vi "FrameToTag(scalar)__slk_mt.vi"(8 "error in (no error)":errorcluster, 10 "frame":string, 11 "string adapter in":refnum<class "StringAdapter__slk_mt.lvclass">) -> (0 "error out":errorcluster, 2 "tag":string, 3 "string adapter out":refnum<class "StringAdapter__slk_mt.lvclass">)   [LabVIEW 2015, in "StringAdapter__slk_mt.lvclass"]
doc: "Converts case frame name to tree control tag."
uses:
  StringAdapter__slk_mt.lvclass
panel:
  # "FrameToTag(scalar)__slk_mt.vi\nConverts case frame name to tree control tag.\n\nNOTICE -- YOU MUST LEAVE THIS NOTICE IN PLACE.\n\nCopyright (c) 2011, LIANG LIU Shawn.Liu.cn@gmail.com\nAll rights reserved.\n\nRedistribution and use in source and binary forms, with or without modification, are permitted provided that the following conditions are met:\n-Redistributions of source code must retain the above copyright notice, this list of conditions and the following disclaimer.\n-Redistributions in binary form must reproduce the above copyright notice, this list of conditions and the following disclaimer in the documentation and/or other materials provided with the distribution.\n-Neither the name of the eLp nor the names of its contributors may be used to endorse or promote products derived from this software without specific prior written permission.\n\nTHIS SOFTWARE IS PROVIDED BY THE COPYRIGHT HOLDERS AND CONTRIBUTORS \"AS IS\" AND ANY EXPRESS OR IMPLIED WARRANTIES, INCLUDING, BUT NOT LIMITED TO, THE IMPLIED WARRANTIES OF MERCHANTABILITY AND FITNESS FOR A PARTICULAR PURPOSE ARE DISCLAIMED. IN NO EVENT SHALL THE COPYRIGHT HOLDER OR CONTRIBUTORS BE LIABLE FOR ANY DIRECT, INDIRECT, INCIDENTAL, SPECIAL, EXEMPLARY, OR CONSEQUENTIAL DAMAGES (INCLUDING, BUT NOT LIMITED TO, PROCUREMENT OF SUBSTITUTE GOODS OR SERVICES; LOSS OF USE, DATA, OR PROFITS; OR BUSINESS INTERRUPTION) HOWEVER CAUSED AND ON ANY THEORY OF LIABILITY, WHETHER IN CONTRACT, STRICT LIABILITY, OR TORT (INCLUDING NEGLIGENCE OR OTHERWISE) ARISING IN ANY WAY OUT OF THE USE OF THIS SOFTWARE, EVEN IF ADVISED OF THE POSSIBILITY OF SUCH DAMAGE."
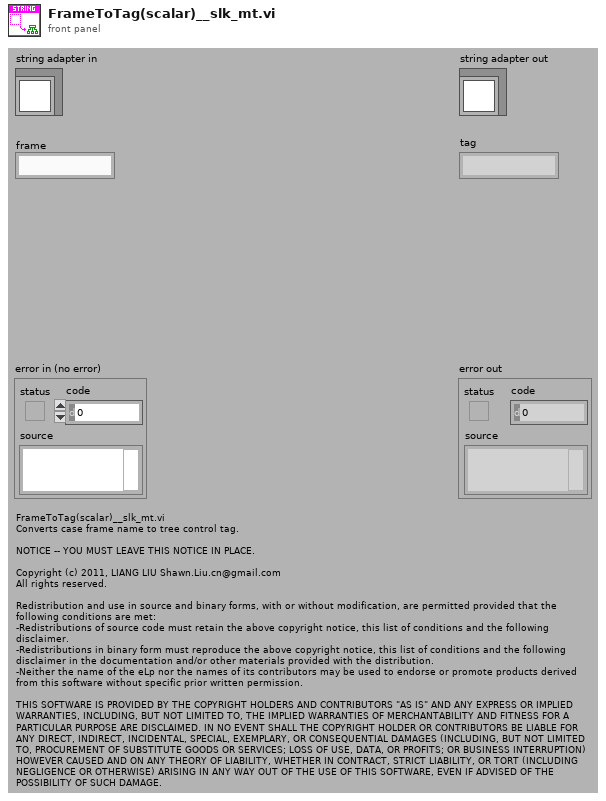
[diagram p1: front panel]
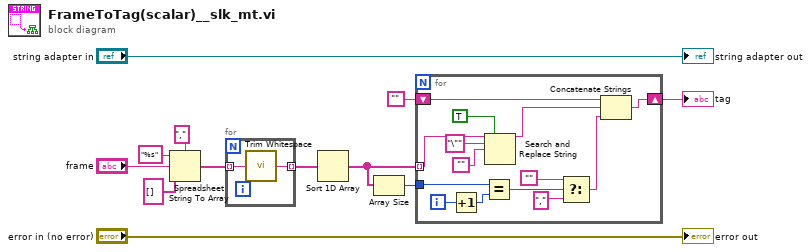
[diagram p0: block diagram]
diagram:
  n1 = Spreadsheet String To Array(delimiter (Tab)="," ("search string"), format string="%s", spreadsheet string="frame", array type (2D Dbl)=string[] []) -> (array=w6:string[])
  n2 = for {
    tunnel: w6 -> [w14] mode=indexing
    tunnel: [w13] -> w5 mode=indexing
    n3 = call <vilib>:"Trim Whitespace.vi"("string"=w14) -> ("trimmed string"=w13:string)  [unwired: 1 in]
  }
  n4 = Sort 1D Array(array=w5) -> (sorted array=w11:string[])
  n5 = Array Size(array=w11) -> (size(s)=w12:i32)
  n6 = for {
    tunnel: w11 -> [w16] mode=indexing
    shift-right: [w28] -> w4
    shift-left: "" -> [w27]
    tunnel: w12 -> [w20]
    i -> [w26]
    n7 = Increment(x=w26) -> (x+1=w25:i32)
    n8 = Equal?(x=w20, y=w25) -> (x = y?=w24:bool)
    n9 = Search and Replace String(replace all?=TRUE ("replace all? (F)"), input string=w16, search string="\"", replace string="") -> (result string=w15:string)  [unwired: 4 in, 3 out]
    n10 = Select(t="", s=w24, f="," ("search string")) -> (s? t:f=w23:string)
    n11 = Concatenate Strings(w27, w15, w23) -> (w28:string)
  }
  "tag" <- w4
  "error out" <- "error in (no error)"
  "string adapter out" <- "string adapter in"
